vi "TEST - Write INI Cluster.vi"(8 "error in (no error)":errorcluster) -> (0 "error out":errorcluster, 2 "Passed":bool)   [LabVIEW 2020]
uses:
  <vilib>/Utility/config.llb/NI_LVConfig.lvlib
  <userlib>/_OpenG.lib/file/file.llb/openg_file.lvlib
  <vilib>/addons/_JKI Toolkits/Caraya/classes/Test/Test.lvclass
  <vilib>/addons/_JKI Toolkits/Caraya/classes/Assert/Assert.lvclass
  <vilib>/addons/_JKI Toolkits/Caraya/classes/Assert/Assert True.vi
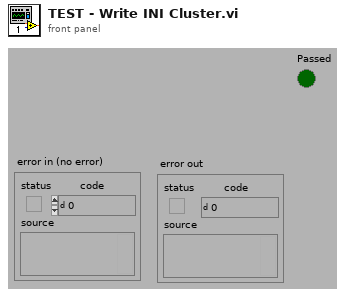
[diagram p1: front panel]
types:
  T1 = cluster{"Section 1":cluster{"Float":dbl, "Integer":i32}, "Section 2":cluster{"Boolean":bool, "String":string}}
  T2 = typedef "NI_LVConfig.lvlib/Config Data RefNum.ctl" = refnum<k1>
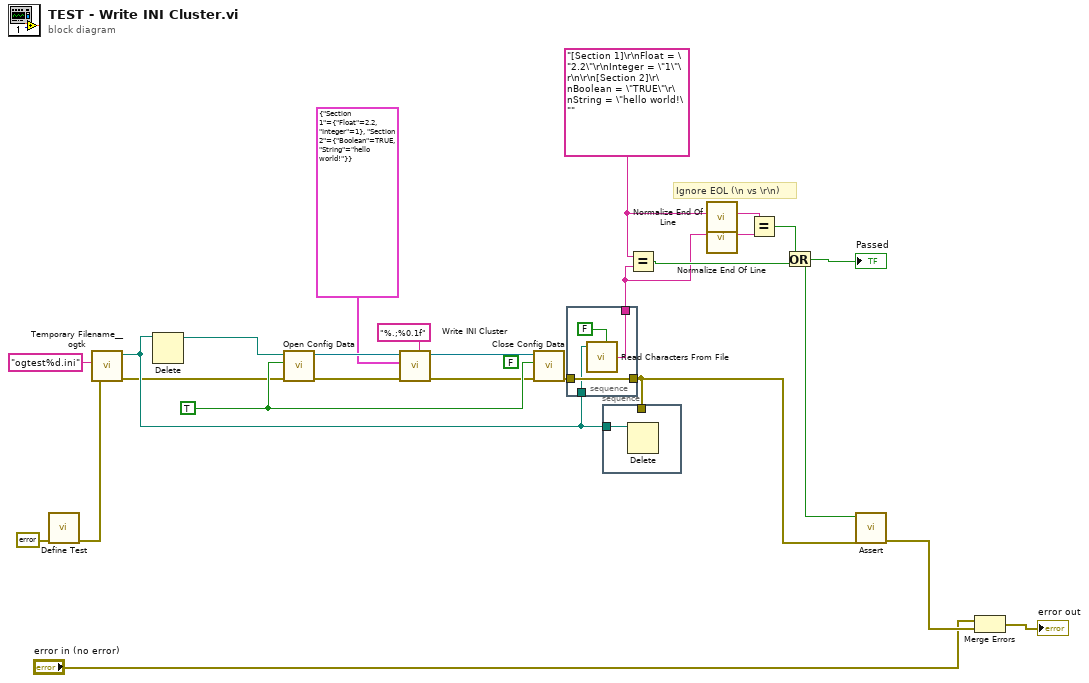
[diagram p0: block diagram]
diagram:
  w5 = "[Section 1]\r\nFloat = \"2.2\"\r\nInteger = \"1\"\r\n\r\n[Section 2]\r\nBoolean = \"TRUE\"\r\nString = \"hello world!\"" ("Display")
  (unwired) FALSE ("write configuration file? (T)")
  w24 = TRUE ("create file if necessary? (T)")
  # "Ignore EOL (\\n vs \\r\\n)"
  n1 = call <vilib>:"Define Test.vi"("error in (no error)"=errorcluster {"status"=FALSE, "code"=0, "source"=""}) -> ("error out"=w10:errorcluster)  [unwired: 9 in, 1 out]
  n2 = call <userlib>:"Temporary Filename__ogtk.vi"("error in (no error)"=w10, "pattern (lvtemp%d.tmp)"="ogtest%d.ini") -> ("error out"=w14:errorcluster, "file in tmp dir"=w15:path)  [unwired: 4 in]
  n3 = Delete(path (use dialog)=w15) -> (deleted path=w22:path)  [unwired: 4 in, 2 out]
  n4 = call <vilib>:"Open Config Data.vi"("error in (no error)"=w14, "create file if necessary (T)"=w24, "configuration file path"=w22) -> ("error out"=w20:errorcluster, "refnum"=w21:T2)  [unwired: 6 in, 1 out]
  n5 = call "Write INI Cluster.vi"("float number format (optional)"="%.;%0.1f", "error in (no error)"=w20, "INI Fomatted Cluster"=T1 {"Section 1"={"Float"=2.2, "Integer"=1}, "Section 2"={"Boolean"=TRUE, "String"="hello world!"}}, "refnum"=w21) -> ("error out"=w23:errorcluster, "dup refnum"=w25:T2)  [unwired: 6 in]
  n6 = call <vilib>:"Close Config Data.vi"("error in (no error)"=w23, "write file if changed (T)"=w24, "refnum"=w25) -> ("error out"=w18:errorcluster)  [unwired: 7 in, 1 out]
  n7 = stacked-sequence {
    tunnel: w18 -> [w29]
    tunnel: [w29] -> w9
    tunnel: w15 -> [w28]
    tunnel: [w27] -> w4
    frame #0 {
      n8 = call <vilib>:"Read Characters From File.vi"("file path (dialog if empty)"=w28, "convert eol? (no:F)"=FALSE) -> ("character string"=w27:string)  [unwired: 4 in, 3 out]
    }
  }
  n9 = stacked-sequence {
    tunnel: w15 -> [w30]
    tunnel: w9 -> [_]
    frame #0 {
      n10 = Delete(path (use dialog)=w30) -> ()  [unwired: 4 in, 3 out]
    }
  }
  n11 = Equal?(x=w5, y=w4) -> (x = y?=w12:bool)
  n12 = call <vilib>:"Normalize End Of Line.vi"("string in"=w5) -> ("string out"=w3:string)  [unwired: 7 in]
  n13 = call <vilib>:"Normalize End Of Line.vi"("string in"=w4) -> ("string out"=w2:string)  [unwired: 7 in]
  n14 = Equal?(x=w3, y=w2) -> (x = y?=w13:bool)
  n15 = Or(x=w13, y=w12) -> (x .or. y?=w1:bool)
  "Passed" <- w1
  n16 = call-poly <vilib>:"Assert.vi"("error in (no error)"=w9, "True?"=w1) -> ("error out"=w8:errorcluster)  [unwired: 8 in, 1 out]
  n17 = Merge Errors("error in (no error)", w8) -> (→"error out":errorcluster)
